vi "ValidateSELECTInputs.vi"(8 "error in (no error)":errorcluster, 10 "columns":string[](array[string]), 11 "table":string) -> (0 "error out":errorcluster, 2 "columns out":string[](array[string]), 3 "table out":string)   [LabVIEW 2019, in "libpqutility.lvlib"]
uses:
  libpqutility.lvlib
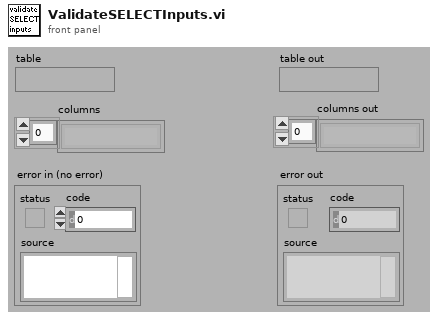
[diagram p1: front panel]
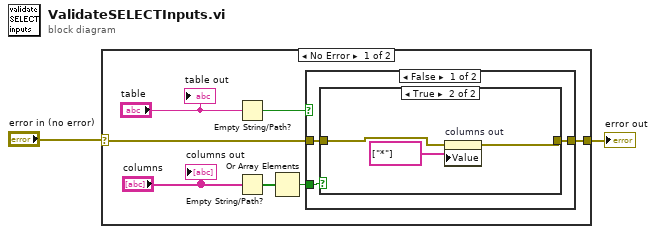
[diagram p0: block diagram]
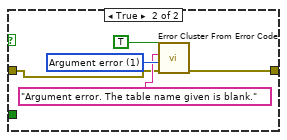
[diagram p3: hidden frame]
diagram:
  n1 = case shown="No Error" "error in (no error)" {
    selector: "error in (no error)" -> [w4 w22]
    tunnel: [w6 w22] -> w2
    frame No Error {
      n2 = Empty String/Path?(string/path="table") -> (empty?=w8:bool)
      n3 = Empty String/Path?(string/path="columns") -> (empty?=w7:bool[])
      n4 = Or Array Elements(Boolean array=w7) -> (logical OR=w9:bool)
      n5 = case shown="False" w8 {
        tunnel: w4 -> [w12 w18]
        tunnel: w9 -> [w10 _]
        tunnel: [w11 w17] -> w6
        frame False {
          n6 = case shown="True" w10 {
            tunnel: w12 -> [w13 w16]
            tunnel: [w13 w14] -> w11
            frame False {
            }
            frame True {
              n7 = property on="columns out" class="Arr (strict)"(error in=w16, "Value"=string[] ["*"] ("columns out")) -> (error out=w14:errorcluster)  [unwired: 1 in, 1 out]
            }
          }
        }
        frame True {
          w20 = 1 items=["No error", "Argument error", "Memory is full", "Out of zone", "End of file", "File already open", "Generic file I/O error", "File not found", "File permission error", "Disk is full", "Duplicate path", "Too many files open", "System feature not enabled", "Resource file not found", "Cannot add resource", "Resource not found", "Image not found", "Image memory error", "Pen does not exist", "Config type invalid", "Config token not found", "Config parse error", "Config memory error", "Bad external code format", "Bad external code offset", "External code not present", "Null window", "Destroy window error", "Null menu", "Print aborted", "Bad print record", "Print driver error", "Windows error during printing", "Memory error during printing", "Print dialog error", "Generic print error", "Invalid device refnum", "Device not found", "Device parameter error", "Device unit error", "Cannot open device", "Device call aborted", "Generic error", "Cancelled by user", "Object ID too low", "Object ID too high", "Object not in heap", "Unknown heap", "Unknown object (invalid DefProc)", "Unknown object (DefProc not in table)", "Message out of range", "Invalid (null) method", "Unknown message", "Manager call not supported", "Bad address", "Network operation in progress", "Network operation timed out", "Connection is busy", "Network attribute not supported", "Network error", "Address in use", "System out of memory", "Connection aborted", "Connection refused", "Not connected", "Already connected", "Connection closed", "Initialization error (interapplication manager)", "Bad occurrence", "Wait on unbound occurrence handler", "Occurrence queue overflow", "Datalog type conflict", "Unused", "Unrecognized type (interapplication manager)", "Memory corrupt", "Failed to make temporary DLL", "Old CIN version", "Drag socket not found", "Failed to load drop-object", "Failed to register OLE object", "Failed to release OLE object", "Format specifier type mismatch", "Unknown format specifier", "Too few format specifiers", "Too many format specifiers", "Scan failed", "Newer CIN version", "Error converting to variant", "Runtime menu error", "Password tampered", "Variant attribute not found", "Incompatible variant data type", "Event data is not available", "Event Store is not present", "Occurrence is not found", "Event Queue is not created", "Event info is not available", "Refnum passed is NULL", "Error retrieving Class GUID", "Error retrieving CoClass GUID", "Error retrieving TypeLib GUID.", ""]
          n8 = call <vilib>:"Error Cluster From Error Code.vi"("show call chain? (False)"=TRUE ("status"), "error in (no error)"=w18, "error message (\"\")"="Argument error. The table name given is blank." ("source"), "error code (0)"=w20) -> ("error out"=w17:errorcluster)  [unwired: 5 in]
        }
      }
      "table out" <- "table"
      "columns out" <- "columns"
    }
    frame Error {
    }
  }
  "error out" <- w2
